vi "Move Axis by Tick.vi"(9 "Tick Scale":dbl, 10 "Axis Focus Value":dbl, 11 "GraphScale in":refnum<vi>) -> ()   [LabVIEW 2021, in "ScrollZoomGraphChart.lvclass"]
uses:
  ScrollZoomGraphChart.lvclass
  ScrollZoomGraphChart.lvclass/ScrollZoomGraphChart.ctl
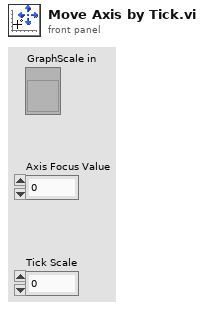
[diagram p1: front panel]
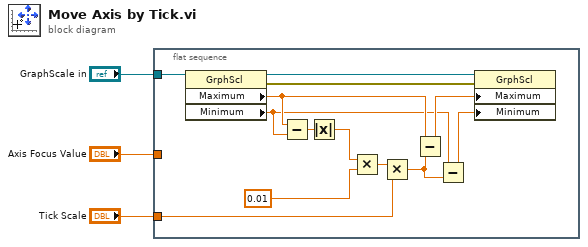
[diagram p0: block diagram]
diagram:
  n1 = flat-sequence {
    tunnel: "Axis Focus Value" -> [_]
    tunnel: "Tick Scale" -> [w6]
    tunnel: "GraphScale in" -> [w13]
    frame #0 {
      n2 = property class="GrphScl"(reference=w13) -> (reference out=w16:refnum<vi>, error out=w12:errorcluster, "Maximum"=w11:dbl, "Minimum"=w8:dbl)  [unwired: 1 in]
      n3 = Subtract(x=w11, y=w8) -> (x-y=w10:dbl)
      n4 = Absolute Value(x=w10) -> (abs(x)=w7:dbl)
      n5 = Multiply(x=w7, y=0.01) -> (x*y=w4:dbl)
      n6 = Multiply(x=w4, y=w6) -> (x*y=w5:dbl)
      n7 = Subtract(x=w11, y=w5) -> (x-y=w15:dbl)
      n8 = Subtract(x=w8, y=w5) -> (x-y=w14:dbl)
      n9 = property class="GrphScl"(reference=w16, error in=w12, "Maximum"=w15, "Minimum"=w14) -> ()  [unwired: 2 out]
    }
  }
